vi "Set Reference Target Name.vi"(10 "Reference Target Name":string, 11 "Project Sync Tools in":refnum<class "Project Sync Tools.lvclass">) -> (3 "Project Sync Tools out":refnum<class "Project Sync Tools.lvclass">)   [LabVIEW 2019, in "Project Sync Tools.lvclass"]
uses:
  Project Sync Tools.lvclass
  Project Sync Tools.lvclass/Project Sync Tools.ctl
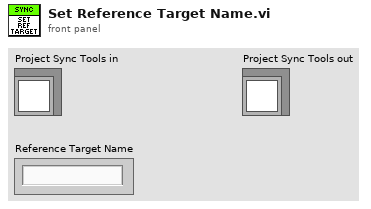
[diagram p1: front panel]
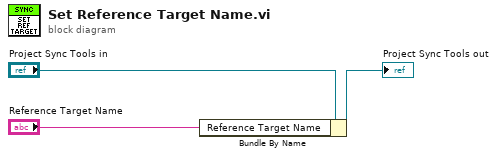
[diagram p0: block diagram]
diagram:
  n1 = Bundle By Name(cluster="Project Sync Tools in", "Reference Target Name"="Reference Target Name") -> (→"Project Sync Tools out":refnum<class "Project Sync Tools.lvclass">)
